vi "Read Task Updated.vi"(8 "error in (no error)":errorcluster, 11 "Task Setting Editor in":refnum<class "Task Setting Editor.lvclass">) -> (0 "error out":errorcluster, 2 "Task Updated":refnum<user-event>, 3 "Task Setting Editor out":refnum<class "Task Setting Editor.lvclass">)   [LabVIEW 2017, in "Task Setting Editor.lvlib" / "Task Setting Editor.lvclass"]
uses:
  Task Setting Editor.lvclass
  BuildWorker/Classes/Task/Task.lvclass
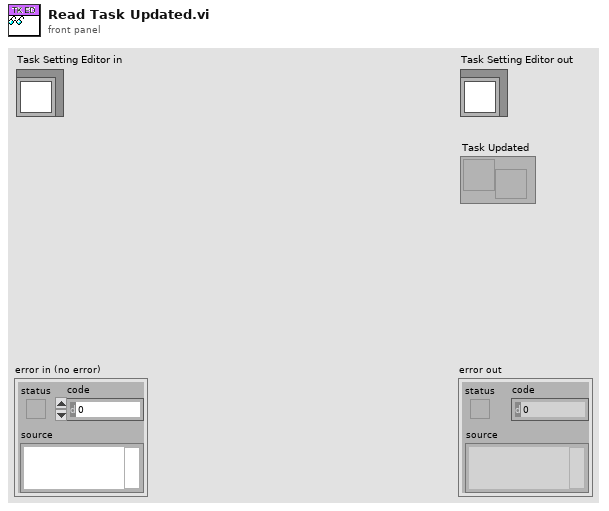
[diagram p1: front panel]
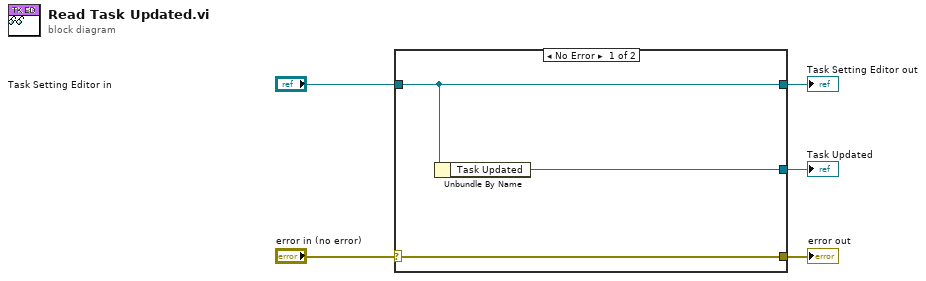
[diagram p0: block diagram]
diagram:
  n1 = case shown="No Error" "error in (no error)" {
    selector: "error in (no error)" -> [w8 w9]
    tunnel: [w8 w9] -> w4
    tunnel: [w7 w10] -> w2
    tunnel: "Task Setting Editor in" -> [w7 w10]
    tunnel: [w6 _] -> w1
    frame No Error {
      n2 = Unbundle By Name(w7) -> ("Task Updated"=w6:refnum<user-event>)
    }
    frame Error {
    }
  }
  "error out" <- w4
  "Task Setting Editor out" <- w2
  "Task Updated" <- w1
